vi "Pendulum get Fw Version.vi"(11 "instance":i32) -> (3 "function return":dbl)   [LabVIEW 2024, in "pendulumApp.lvlib"]
doc: "OOTB_API double Pendulum_getFwVersion();\n\nOOTB_API double Pendulum_getFwVersion(int instance);"
uses:
  pendulumApp.lvlib
  pendulumApp.dll
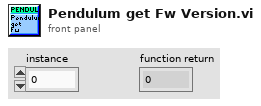
[diagram p1: front panel]
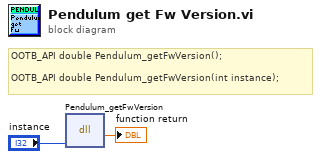
[diagram p0: block diagram]
diagram:
  # "OOTB_API\tdouble Pendulum_getFwVersion();\n\nOOTB_API\tdouble Pendulum_getFwVersion(int instance);"
  n1 = dll-call lib="C:/Users/scer/OneDrive - University of Florida/eml4314c/eml4314cFA25/Resources/FA25_dev_version2/SADI_Pendulum_lib/pendulumApp.*" fn="Pendulum_getFwVersion"("instance"="instance") -> (→"function return":dbl)  [unwired: 4 in, 2 out]
